vi "MicroscopeActor.vi"(8 "error in (no error)":errorcluster) -> (0 "error out":errorcluster)   [LabVIEW 2017]
doc: "Use this template to build a VI to use as a subVI."
uses:
  Spectrometer Utilities/SpectrometerCallbackdataEvent.ctl
  Microscope/MicroscopeControllerCluster.ctl
  <vilib>/vision/Image Controls.llb/IMAQ Image.ctl
  Microscope/MicroscopeActorCluster.ctl
  Database/DatabaseContollerGFVenum.ctl
  Microscope/MicroscopeControllerEnum.ctl
  <vilib>/userdefined/High Color/IMAQdx.ctl
  <vilib>/vision/driver/IMAQdx.llb/IMAQdx Camera Control Mode.ctl
  <vilib>/event_ctls.llb/lveventtype.ctl
  <vilib>/vision/NI_Vision_Development_Module.lvlib
  <vilib>/vision/driver/NI_Vision_Acquisition_Software.lvlib
panel:
  in  "Microscope Objective":u16(ring) caption="Combo Box" items=["50x", "5x", "10x"]
  in  "micron/pixel":dbl=0.10791300237178802
  in  "user event out":refnum<user-event>
  in  "user event Callback":refnum<user-event>
  in  "Add Objective":bool
  in  "TabEncompassingEditPointsControls":enum32{"Page 2"}(tab)
  in  "Choose Points":enum32{"Edit map Points", "Edit Laser Point"}(radio)=enum."Edit Laser Point"
  in  "TabEncompassMapEditControls":enum32{"Page 2"}(tab)
  in  "UndoBtn":bool
  out "# Points Selected":i32
  in  "Point Spacing":dbl=1.0 min=0.5 max=1000.0 format="%#_g µm"
  in  "Clear Points":bool
  in  "Edit Points":bool
  in  "Edit Laser Position":bool
  in  "Edit Map Points":bool=TRUE
  in  "Which point to translate?":i32
  in  "stop":bool
  out "Microscope Image":T1(plugin-control)
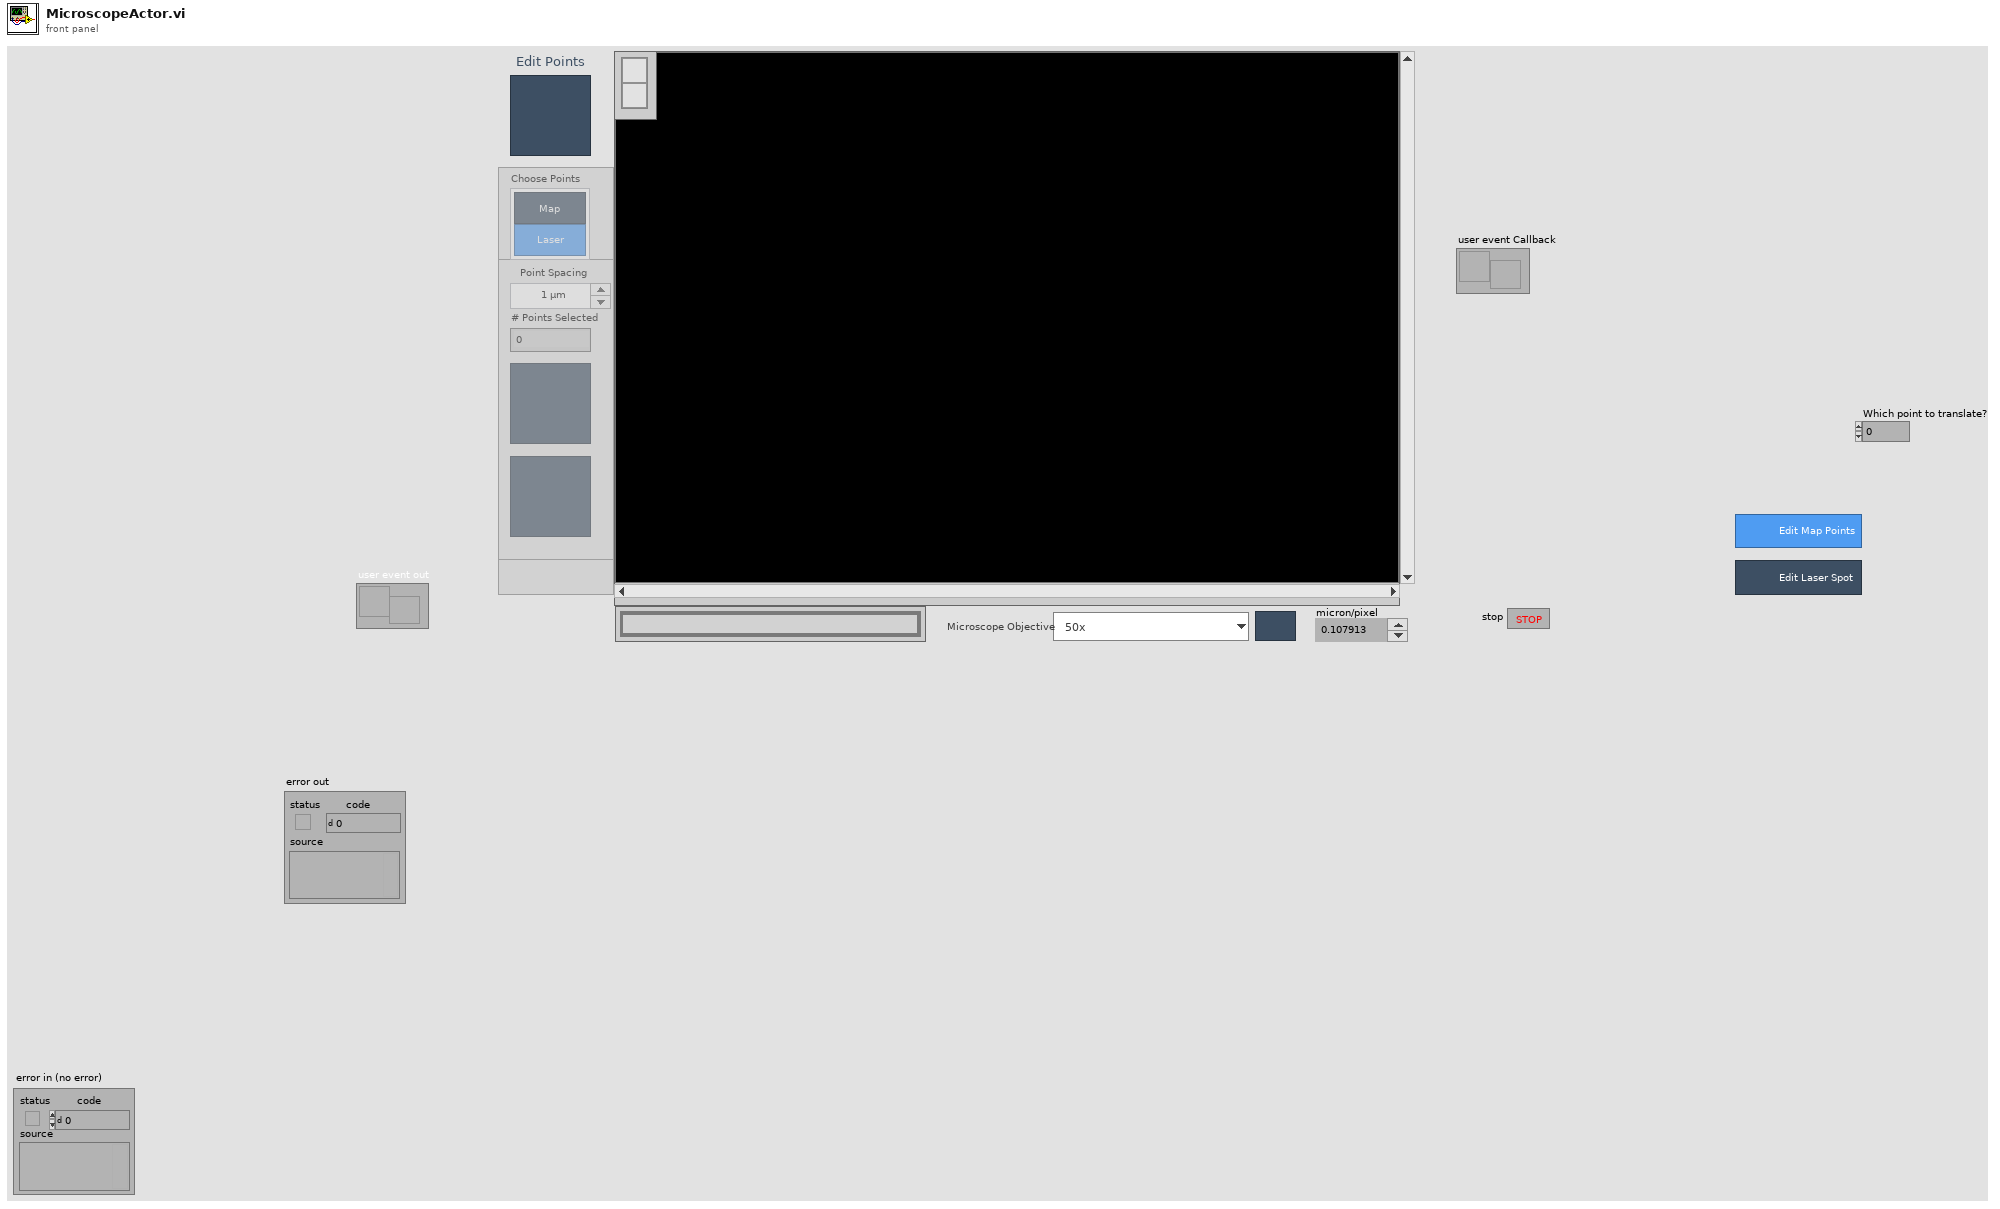
[diagram p1: front panel]
types:
  T1 = typedef "IMAQ Image.ctl" = refnum<image>
  T2 = typedef "Image Type" = u32
  T3 = typedef "DatabaseContollerGFVenum.ctl" = enum16{"Init and Open Database!", "GetTimeDifferencebetweenLastTwoMeasurements!", "Get next Journal Number!", "WriteInJournalTable", "GetNewMeas_dataIndex", "UpdateWithSpectrometerData", "UpdateWithMicroscopeData", "UpdateWithMapScriptData", "UpdateWithmainUIData", "Get Objective Microns/Pixels", "Get User Name!", "Get Active Users Names!", "Get User Picture!", "Get User Phone Number!", "Get Setup Names!", "Get Active Microscope Objectives!", "Get Experiment Number!", "Get Sample Types!", "Write meas_conf Table", "Write meas_data Table", "GetListOfIndices", "Get Objective Index", "Get last X Journal Entries"}
  T4 = typedef "MicroscopeControllerEnum.ctl" = enum16{"GetAllData!", "Init!", "Start!", "Stop!", "GetMicroscopeVIRef", "CalculateRelPointForStagemicrons", "InsertCallbackEvent!", "InsertLaserPoint!", "InsertMapPoints!", "InsertMicroscopeOverlayImageRef!", "GetMicroscopeOverlayImageRef", "InsertObjectiveIndex!", "InsertLiveImageRef", "GetLiveImageRef"}
  T5 = typedef "Image Unit" = enum32{"Undefined", "Angström", "Micrometer", "Millimeter", "Centimeter", "Meter", "Kilometer", "Microinch", "Inch", "Feet", "Nautical miles", "Standard miles", "Steps"}
  T6 = typedef "Simple Grid Descriptor" = cluster{"X Step":sgl, "Y Step":sgl, "Unit":T5}
  T7 = typedef "NI_Vision_Acquisition_Software.lvlib/IMAQdx Camera Control Mode.ctl" = enum32{"Controller", "Listener"}
  T8 = typedef "IMAQdx.ctl" = refnum<k21>
  T9 = typedef "MicroscopeActorCluster.ctl" = cluster{"Calibration Axis ":cluster{"Origin Pixel":cluster{"X":sgl, "Y":sgl}, "Angle Relative to Horizontal (deg)":sgl, "Axis Reference":u32}, "Microscope Image Overlay Ref":T1, "Laser Coordinate":cluster{"X":i32, "Y":i32}, "Map Points Coordinates":cluster{"X":i32, "Y":i32}[], "micron/pixel":dbl, "Microscope Image Live Ref":T1}
  T10 = cluster{"Origin Pixel":cluster{"X":sgl, "Y":sgl}, "Angle Relative to Horizontal (deg)":sgl, "Axis Reference":u32}
  T11 = typedef "MicroscopeControllerCluster.ctl" = cluster{"MapPointsArray":cluster{"X":i32, "Y":i32}[], "Laser Point Coor":cluster{"X":i32, "Y":i32}, "Microscope Image Overlay Ref":T1, "idObjectives":u32, "Microscope Image Live":T1}
  T12 = typedef "lveventtype.ctl" = enum32{"Null", "Timeout", "Annotation Menu Selection", "Annotation Menu Selection?", "App Instance Close", "App Instance Close?", "Autoscale Range Change", "Bookmark Info Change", "Cell Edit", "Cell Edit?", "Cursor Grab", "Cursor Grab?", "Cursor Menu Selection", "Cursor Menu Selection?", "Cursor Move", "Cursor Release", "Data Change", "Direction Change", "Display State Change", "Drag Ended", "Drag Enter", "Drag Leave", "Drag Over", "Drag Source Update", "Drag Starting", "Drag Starting?", "Drop", "Exec State Change", "Key Down", "Key Down?", "Key Repeat", "Key Repeat?", "Key Up", "Listbox Double Click", "Menu Activation?", "Menu Selection (App)", "Menu Selection? (App)", "Menu Selection (User)", "Mouse Down", "Mouse Down?", "Mouse Enter", "Mouse Leave", "Mouse Move", "Mouse Up", "Mouse Wheel", "NI Security User Change (App)", "Pane Size", "Panel Close", "Panel Close?", "Panel Resize", "Plot Attribute Change", "Scale Range Change", "Shortcut Menu Activation?", "Shortcut Menu Selection (App)", "Shortcut Menu Selection? (App)", "Shortcut Menu Selection (User)", "Tree Double Click", "Tree Drag", "Tree Drag?", "Tree Drop", "Tree Drop?", "Tree Item Close", "Tree Item Close?", "Tree Item Open", "Tree Item Open?", "User Event", "Value Change"}
  T13 = cluster{"Left":i32, "Top":i32, "Right":i32, "Bottom":i32}
  T14 = enum8{"Enabled", "Disabled", "Disabled and Grayed Out"}
  T15 = cluster{"Global Rectangle":i32[], "Contours":cluster{"Contour Type":u32, "ROI Type":u32, "Points":i32[]}[]}
  T16 = cluster{"Contour Type":u32, "ROI Type":u32, "Points":i32[]}[]
  T17 = cluster{"Contour Type":u32, "ROI Type":u32, "Points":i32[]}
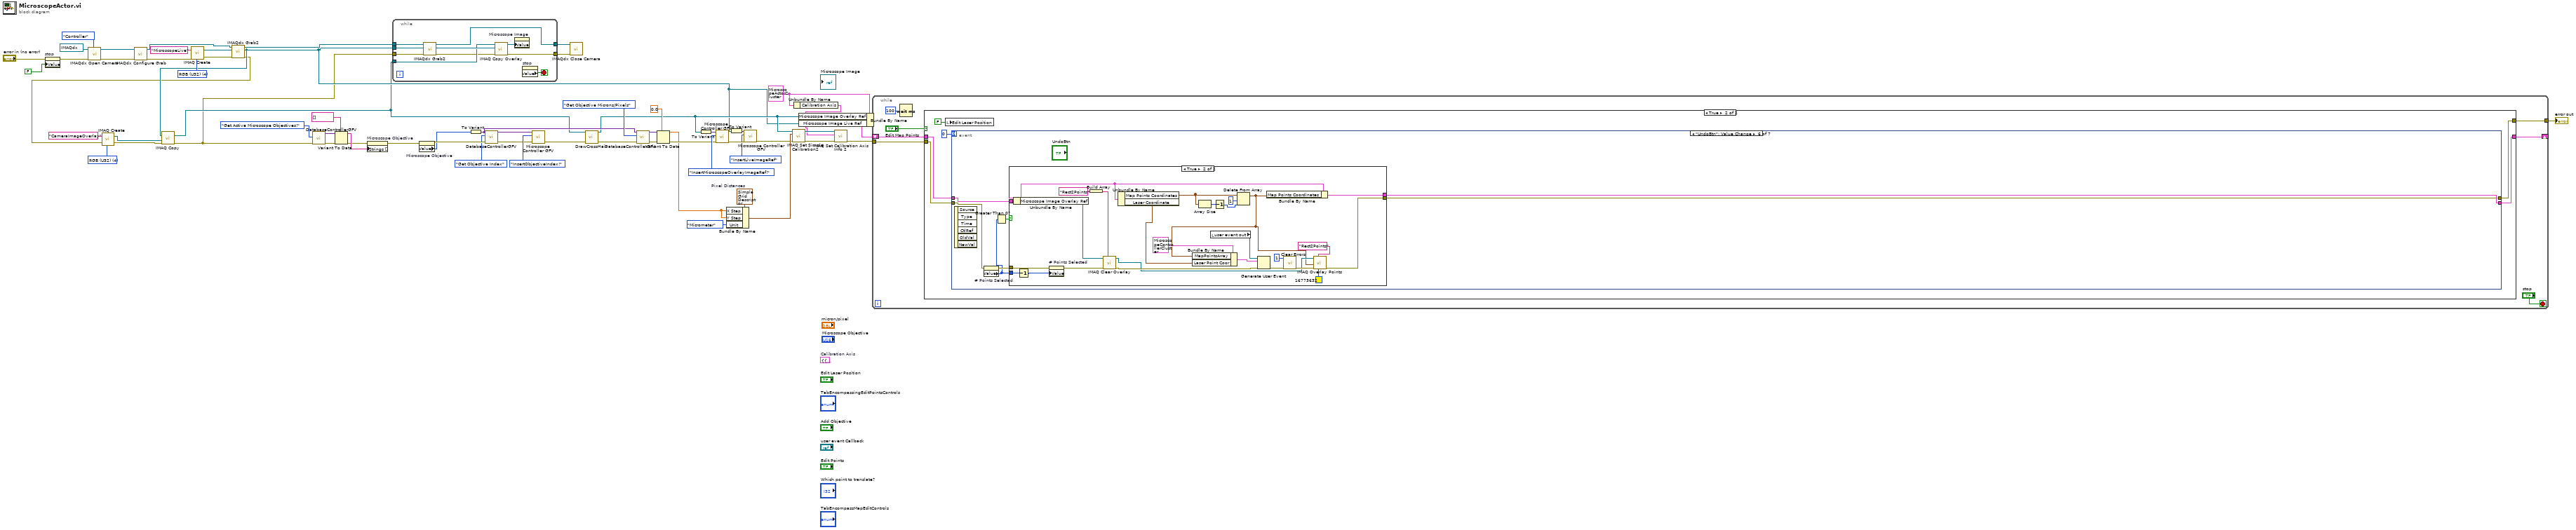
[diagram p0: block diagram]
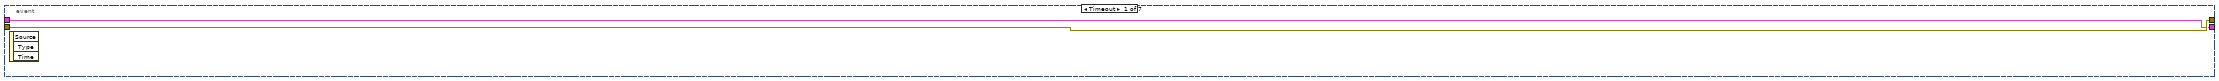
[diagram p3: hidden frame]
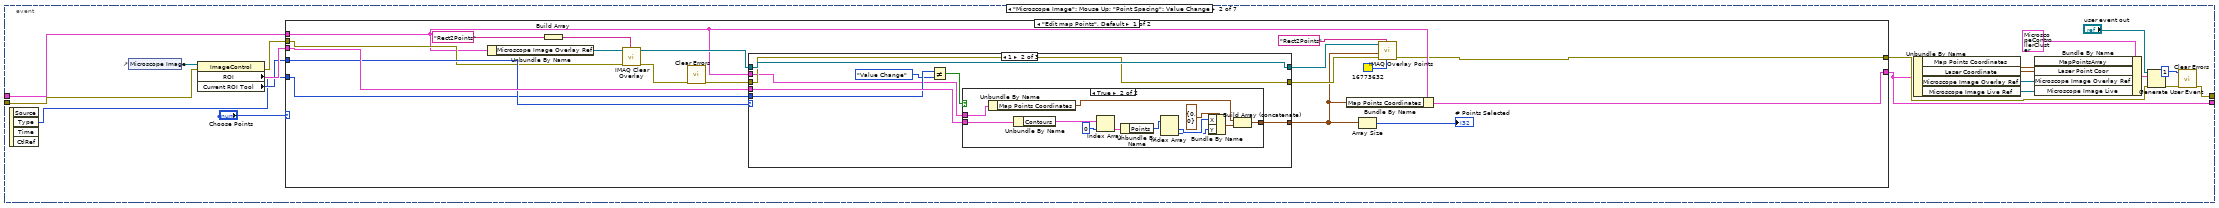
[diagram p4: hidden frame]
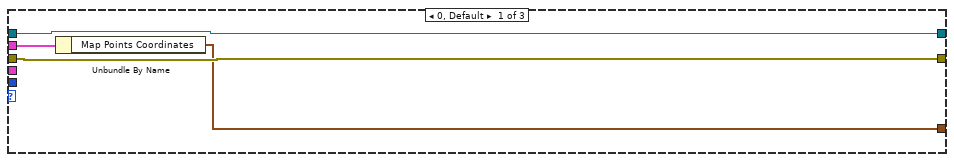
[diagram p5: hidden frame]
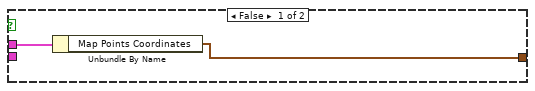
[diagram p6: hidden frame]
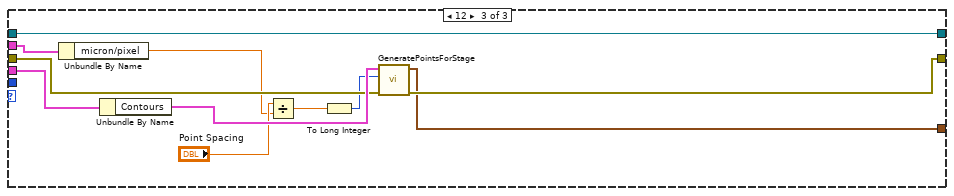
[diagram p7: hidden frame]
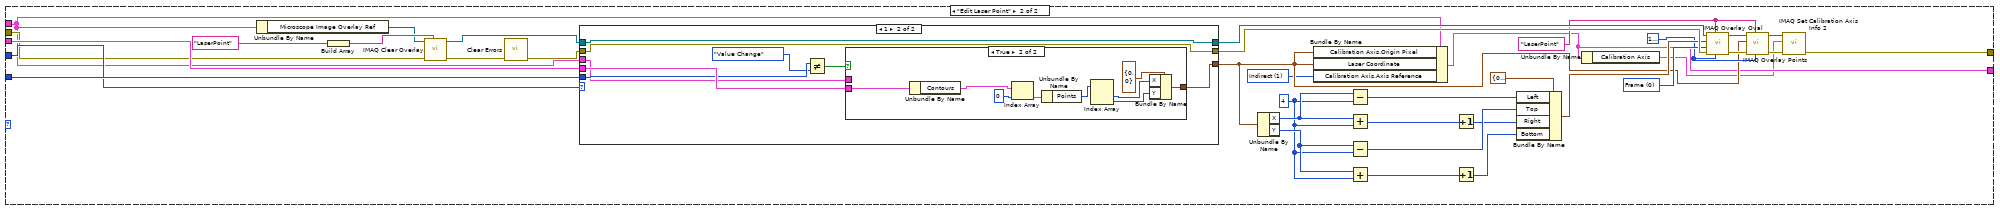
[diagram p8: hidden frame]
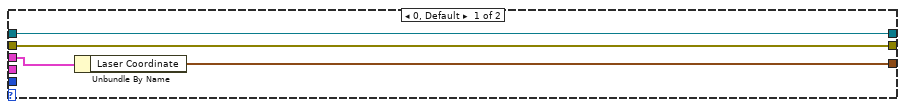
[diagram p9: hidden frame]
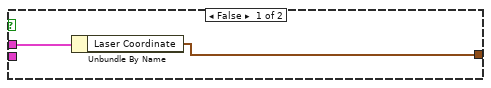
[diagram p10: hidden frame]
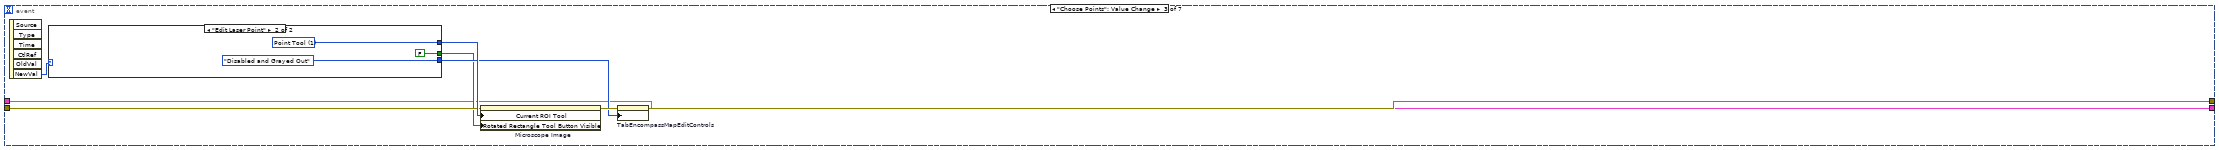
[diagram p11: hidden frame]
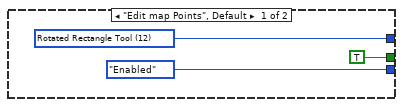
[diagram p12: hidden frame]
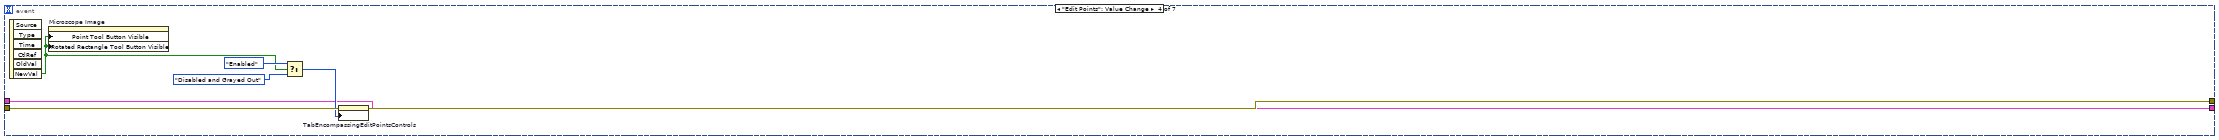
[diagram p13: hidden frame]
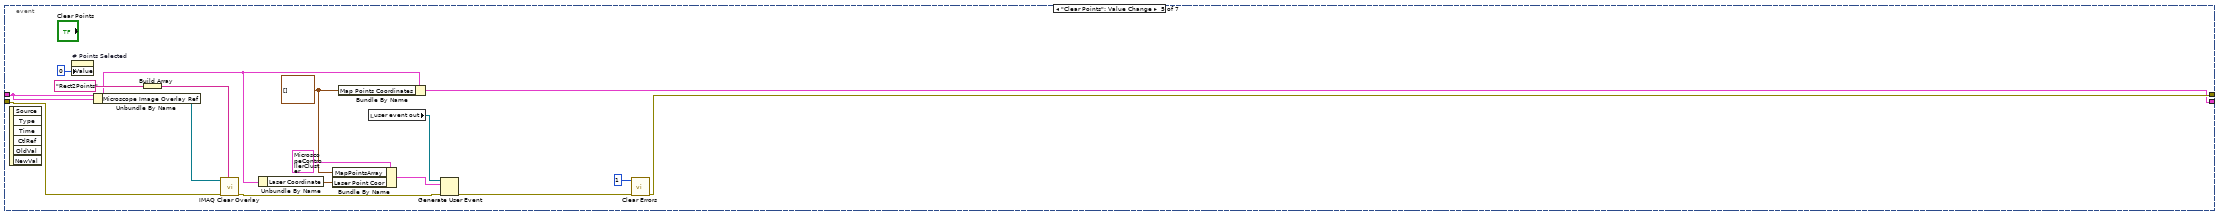
[diagram p14: hidden frame]
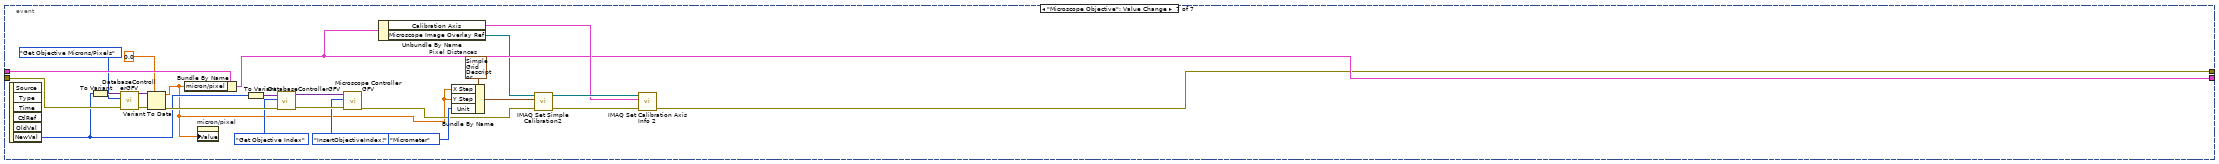
[diagram p16: hidden frame]
diagram:
  w15 = T2 4 items=["Grayscale (U8)", "Grayscale (I16)", "Grayscale (SGL)", "Complex (CSG)", "RGB (U32)", "HSL (U32)", "RGB (U64)", "Grayscale (U16)"] ("Image Type")
  w37 = T2 4 items=["Grayscale (U8)", "Grayscale (I16)", "Grayscale (SGL)", "Complex (CSG)", "RGB (U32)", "HSL (U32)", "RGB (U64)", "Grayscale (U16)"] ("Image Type")
  w45 = T6 {"X Step"=0.08029388, "Y Step"=0.08029388, "Unit"=enum."Micrometer"}  # Pixel Distances
  w39 = T9 {"Calibration Axis "={"Origin Pixel"={"X"=1232.0, "Y"=1028.0}, "Angle Relative to Horizontal (deg)"=0.0, "Axis Reference"=0}, "Microscope Image Overlay Ref"=refnum, "Laser Coordinate"={"X"=0, "Y"=0}, "Map Points Coordinates"=[], "micron/pixel"=0.10791300237178802, "Microscope Image Live Ref"=refnum}
  (unwired) T10 {"Origin Pixel"={"X"=1232.0, "Y"=1028.0}, "Angle Relative to Horizontal (deg)"=0.0, "Axis Reference"=0}  # Calibration Axis
  n1 = property on="stop" class="Bool (strict)"(error in="error in (no error)", "Value"=FALSE ("stop")) -> (error out=w3:errorcluster)  [unwired: 1 in, 1 out]
  n2 = call <vilib>:"IMAQdx Open Camera.vi"("Camera Control Mode"=IMAQdx_Camera_Control_Mode."Controller", "error in"=w3, "Session In"=T8 "cam2") -> ("error out"=w20:errorcluster, "Session Out"=w48:T8)  [unwired: 7 in]
  n3 = call <vilib>:"IMAQdx Configure Grab.vi"("error in"=w20, "Session In"=w48) -> ("error out"=w16:errorcluster, "Session Out"=w9:T8)  [unwired: 8 in]
  n4 = call "IMAQ Create"("Image Name"="MicroscopeLive", "Image Type"=w15, "error in (no error)"=w16) -> ("New Image"=w10:T1, "error out"=w11:errorcluster)  [unwired: 2 in]
  n5 = call <vilib>:"IMAQdx Grab2.vi"("error in"=w11, "Image In"=w10, "Session In"=w9) -> ("error out"=w2:errorcluster, "Image Out"=w5:T1, "Session Out"=w8:T8)  [unwired: 5 in, 1 out]
  n6 = call "IMAQ Create"("Image Name"="CameraImageOverlay", "Image Type"=w37, "error in (no error)"=w2) -> ("New Image"=w6:T1, "error out"=w7:errorcluster)  [unwired: 2 in]
  n7 = call "IMAQ Copy"("error in (no error)"=w7, "Image Dst"=w6, "Image Src"=w5) -> ("error out"=w1:errorcluster, "Image Dst Out"=w4:T1)  [unwired: 3 in]
  n8 = call "DatabaseControllerGFV.vi"("error in (no error)"=w1, "Enum"=DatabaseContollerGFVenum."Get Active Microscope Objectives!") -> ("error out"=w62:errorcluster, "Data Out"=w61:variant)  [unwired: 8 in]
  n9 = Variant To Data(error in=w62, type=string[] [], Variant=w61) -> (data=w59:string[], error out=w58:errorcluster)
  n10 = property on="Microscope Objective" class="Ring (strict)"(error in=w58, "Strings []"=w59) -> (error out=w52:errorcluster)  [unwired: 1 in, 1 out]
  n11 = while {
    tunnel: w8 -> [w73]
    tunnel: [w71] -> w19
    tunnel: [w70] -> w18
    tunnel: w5 -> [w72]
    tunnel: w4 -> [w67]
    tunnel: w1 -> [w64]
    stop <- w65 stop-if-true
    n12 = call <vilib>:"IMAQdx Grab2.vi"("error in"=w64, "Image In"=w72, "Session In"=w73) -> ("error out"=w66:errorcluster, "Image Out"=w69:T1, "Session Out"=w71:T8)  [unwired: 5 in, 1 out]
    n13 = call "IMAQ Copy Overlay"("error in (no error)"=w66, "Image Dst"=w69, "Image Src"=w67) -> ("error out"=w70:errorcluster, "Image Dst Out"=w68:T1)  [unwired: 7 in]
    n14 = property on="Microscope Image" class="ImageControl"("Value"=w68) -> ()  [unwired: 2 in, 2 out]
    n15 = property on="stop" class="Bool (strict)"() -> ("Value"=w65:bool)  [unwired: 2 in, 2 out]
  }
  n16 = property on="Microscope Objective" class="Ring (strict)"(error in=w52) -> (error out=w53:errorcluster, "Value"=w51:u16)  [unwired: 1 in, 1 out]
  n17 = To Variant(anything=w51) -> (Variant=w22:variant)
  n18 = call "DatabaseControllerGFV.vi"("error in (no error)"=w53, "Enum"=DatabaseContollerGFVenum."Get Objective Index", "Data in"=w22) -> ("error out"=w55:errorcluster, "Data Out"=w54:variant)  [unwired: 7 in]
  n19 = call "Microscope Controller GFV.vi"("error in (no error)"=w55, "MicroscopeEnum"=MicroscopeControllerEnum."InsertObjectiveIndex!", "Data in"=w54) -> ("error out"=w14:errorcluster)  [unwired: 7 in, 1 out]
  n20 = call <vilib>:"IMAQdx Close Camera.vi"("error in"=w18, "Session In"=w19) -> ()  [unwired: 9 in, 1 out]
  n21 = call "DrawCrossHair.vi"("error in (no error)"=w14, "Image In"=w4) -> ("error out"=w13:errorcluster, "Image Out"=w12:T1)  [unwired: 8 in]
  n22 = call "DatabaseControllerGFV.vi"("error in (no error)"=w13, "Enum"=DatabaseContollerGFVenum."Get Objective Microns/Pixels", "Data in"=w22) -> ("error out"=w26:errorcluster, "Data Out"=w23:variant)  [unwired: 7 in]
  n23 = Variant To Data(error in=w26, type=0.0 ("data"), Variant=w23) -> (data=w21:dbl, error out=w25:errorcluster)
  n24 = To Variant(anything=w12) -> (Variant=w30:variant)
  n25 = call "Microscope Controller GFV.vi"("error in (no error)"=w25, "MicroscopeEnum"=MicroscopeControllerEnum."InsertMicroscopeOverlayImageRef!", "Data in"=w30) -> ("error out"=w35:errorcluster)  [unwired: 7 in, 1 out]
  n26 = Bundle By Name(cluster=w45, "X Step"=w21, "Y Step"=w21, "Unit"=Image_Unit."Micrometer") -> (w43:T6)
  n27 = To Variant(anything=w5) -> (Variant=w31:variant)
  n28 = call "Microscope Controller GFV.vi"("error in (no error)"=w35, "MicroscopeEnum"=MicroscopeControllerEnum."InsertLiveImageRef", "Data in"=w31) -> ("error out"=w34:errorcluster)  [unwired: 7 in, 1 out]
  n29 = call "IMAQ Set Simple Calibration2"("error in (no error)"=w34, "Pixel Distances"=w43, "Image"=w12) -> ("error out"=w42:errorcluster, "Calibration Template Image"=w40:T1)  [unwired: 7 out]
  n30 = Unbundle By Name(w39) -> ("Calibration Axis"=w38:T10)
  n31 = Bundle By Name(cluster=w39, "Microscope Image Overlay Ref"=w12, "Microscope Image Live Ref"=w5) -> (w46:T9)
  n32 = call-poly "IMAQ Set Calibration Axis Info 2"("error in (no error)"=w42, "Calibration Axis Info"=w38, "Calibration Template Image In"=w40) -> ("error out"=w41:errorcluster)  [unwired: 7 in, 1 out]
  n33 = while {
    tunnel: [w79] -> w63
    tunnel: w41 -> [w78]
    shift-right: [w74] -> _
    shift-left: w46 -> [w75]
    stop <- "stop" stop-if-true
    n34 = Wait (ms)(milliseconds to wait=u32 100) -> ()  [unwired: 1 out]
    n35 = case shown="True" "Edit Map Points" {
      tunnel: [w82 w87] -> w79
      tunnel: w78 -> [w82 w86]
      tunnel: w75 -> [w81 w84]
      tunnel: [w81 w83] -> w74
      frame False {
      }
      frame True {
        n36 = local write "Edit Laser Position"(FALSE ("Edit Laser Position")) -> ()
        n37 = event shown="[5] \"UndoBtn\": Value Change" {
          selector: _ -> [_ _ _ _ _ _ _]
          dyn-events: _ -> [_ _ _ _ _ _ _]
          timeout: 0 -> [_ _ _ _ _ _ _]
          tunnel: [w90 w100 w229 w242 w254 w268 w298] -> w87
          tunnel: w86 -> [w90 w109 w231 w246 w262 w265 w316]
          tunnel: w84 -> [w89 w96 w226 w240 w248 w267 w322]
          tunnel: [w89 w95 w226 w240 w249 w269 w300] -> w83
          event Timeout {
            n38 = event-data() -> ()  [unwired: 1 in, 3 out]
          }
          event "Microscope Image": Mouse Up; "Point Spacing": Value Change {
            n39 = event-data() -> ("Type"=w106:T12)  [unwired: 1 in, 3 out]
            n40 = control-ref of="Microscope Image"() -> (w107:refnum<vi>)
            n41 = property class="ImageControl"(reference=w107, error in=w109) -> (error out=w104:errorcluster, "ROI"=w110:T15, "Current ROI Tool"=w108:u32)  [unwired: 1 out]
            n42 = case shown="\"Edit map Points\", Default" "Choose Points" {
              tunnel: w110 -> [w129 w201]
              tunnel: w108 -> [w128 w200]
              tunnel: w106 -> [w122 w202]
              tunnel: [w111 w167] -> w102
              tunnel: w104 -> [w121 w196]
              tunnel: w96 -> [w112 w175]
              tunnel: [w113 w171] -> w95
              frame "Edit map Points", Default {
                n43 = Unbundle By Name(w112) -> ("Microscope Image Overlay Ref"=w115:T1)
                n44 = Build Array("Rect2Points" ("Group")) -> (w118:string[])
                n45 = call "IMAQ Clear Overlay"("Groups"=w118, "error in (no error)"=w121, "Image"=w115) -> ("error out"=w117:errorcluster, "Image Out"=w120:T1)  [unwired: 7 in]
                n46 = call <vilib>:"Clear Errors.vi"("error in (no error)"=w117) -> ("error out"=w116:errorcluster)  [unwired: 5 in, 1 out]
                n47 = case shown="1" w128 {
                  tunnel: w129 -> [_ w141 w166]
                  tunnel: [w130 w140 w158] -> w114
                  tunnel: [w133 w139 w162] -> w124
                  tunnel: w116 -> [w132 w138 w164]
                  tunnel: w120 -> [w133 w139 w162]
                  tunnel: [w132 w138 w163] -> w126
                  tunnel: w122 -> [_ w137 _]
                  tunnel: w112 -> [w131 w134 w157]
                  frame 0, Default {
                    n48 = Unbundle By Name(w131) -> ("Map Points Coordinates"=w130:cluster{"X":i32, "Y":i32}[])
                  }
                  frame 1 {
                    n49 = Not Equal?(x=w137, y=lveventtype."Value Change" ("Type")) -> (x != y?=w135:bool)
                    n50 = case shown="True" w135 {
                      tunnel: w141 -> [_ w155]
                      tunnel: [w143 w145] -> w140
                      tunnel: w134 -> [w142 w144]
                      frame False {
                        n51 = Unbundle By Name(w142) -> ("Map Points Coordinates"=w143:cluster{"X":i32, "Y":i32}[])
                      }
                      frame True {
                        n52 = Unbundle By Name(w144) -> ("Map Points Coordinates"=w146:cluster{"X":i32, "Y":i32}[])
                        n53 = Unbundle By Name(w155) -> ("Contours"=w154:T16)
                        n54 = Index Array(array=w154, index=0) -> (element=w152:T17)
                        n55 = Unbundle By Name(w152) -> ("Points"=w150:i32[])
                        n56 = Index Array(array=w150) -> (element #1=w149:i32, element #2=w148:i32)  [unwired: 2 in]
                        n57 = Bundle By Name(cluster=cluster{"X":i32, "Y":i32} {"X"=0, "Y"=0} ("Point Coordinates"), "X"=w149, "Y"=w148) -> (w147:cluster{"X":i32, "Y":i32})
                        n58 = Build Array (concatenate)(w146, w147) -> (w145:cluster{"X":i32, "Y":i32}[])
                      }
                    }
                  }
                  frame 12 {
                    n59 = Unbundle By Name(w157) -> ("micron/pixel"=w156:dbl)
                    n60 = Unbundle By Name(w166) -> ("Contours"=w165:T16)
                    n61 = Divide(x="Point Spacing", y=w156) -> (x/y=w160:dbl)
                    n62 = To Long Integer(number=w160) -> (32bit integer=w159:i32)
                    n63 = call "GeneratePointsForStage.vi"("error in (no error)"=w164, "Point Spacing"=w159, "Rotated Rect"=w165) -> ("error out"=w163:errorcluster, "PointsInRotatedRect"=w158:cluster{"X":i32, "Y":i32}[])  [unwired: 7 in]
                  }
                }
                n64 = Bundle By Name(cluster=w112, "Map Points Coordinates"=w114) -> (w113:T9)
                n65 = Array Size(array=w114) -> (size(s)=→"# Points Selected":i32)
                n66 = call "IMAQ Overlay Points"("Color"=u32 16773632, "Group"="Rect2Points", "error in (no error)"=w126, "Array of Points"=w114, "Image"=w124) -> ("error out"=w111:errorcluster)  [unwired: 5 in, 1 out]
              }
              frame "Edit Laser Point" {
                w169 = u32 1 items=["Direct", "Indirect"] ("Axis Reference")
                w177 = 4 ("Laser Spot Size")
                w186 = u32 0 items=["Frame", "Fill"] ("Drawing Mode (Frame)")
                w183 = "LaserPoint" ("Group")
                w184 = u32 16777222 ("Color")
                n67 = Unbundle By Name(w175) -> ("Microscope Image Overlay Ref"=w176:T1)
                n68 = Build Array("LaserPoint" ("Group")) -> (w195:string[])
                n69 = call "IMAQ Clear Overlay"("Groups"=w195, "error in (no error)"=w196, "Image"=w176) -> ("error out"=w193:errorcluster, "Image Out"=w197:T1)  [unwired: 7 in]
                n70 = call <vilib>:"Clear Errors.vi"("error in (no error)"=w193) -> ("error out"=w192:errorcluster)  [unwired: 5 in, 1 out]
                n71 = case shown="1" w200 {
                  tunnel: w201 -> [_ w214]
                  tunnel: [w206 w213] -> w198
                  tunnel: w192 -> [w205 w212]
                  tunnel: w197 -> [w206 w213]
                  tunnel: [w205 w212] -> w199
                  tunnel: w202 -> [_ w211]
                  tunnel: [w203 w208] -> w174
                  tunnel: w175 -> [w204 w207]
                  frame 0, Default {
                    n72 = Unbundle By Name(w204) -> ("Laser Coordinate"=w203:cluster{"X":i32, "Y":i32})
                  }
                  frame 1 {
                    n73 = Not Equal?(x=w211, y=lveventtype."Value Change" ("Type")) -> (x != y?=w209:bool)
                    n74 = case shown="True" w209 {
                      tunnel: w214 -> [_ w225]
                      tunnel: [w215 w217] -> w208
                      tunnel: w207 -> [w216 _]
                      frame False {
                        n75 = Unbundle By Name(w216) -> ("Laser Coordinate"=w215:cluster{"X":i32, "Y":i32})
                      }
                      frame True {
                        n76 = Unbundle By Name(w225) -> ("Contours"=w224:T16)
                        n77 = Index Array(array=w224, index=0) -> (element=w222:T17)
                        n78 = Unbundle By Name(w222) -> ("Points"=w220:i32[])
                        n79 = Index Array(array=w220) -> (element #1=w219:i32, element #2=w218:i32)  [unwired: 2 in]
                        n80 = Bundle By Name(cluster=cluster{"X":i32, "Y":i32} {"X"=0, "Y"=0} ("Point Coordinates"), "X"=w219, "Y"=w218) -> (w217:cluster{"X":i32, "Y":i32})
                      }
                    }
                  }
                }
                n81 = Unbundle By Name(w174) -> ("X"=w188:i32, "Y"=w189:i32)
                n82 = Bundle By Name(cluster=w175, "Calibration Axis.Origin Pixel"=w174, "Laser Coordinate"=w174, "Calibration Axis.Axis Reference"=w169) -> (w171:T9)
                n83 = Subtract(x=w188, y=w177) -> (x-y=w190:i32)
                n84 = Add(x=w188, y=w177) -> (x+y=w178:i32)
                n85 = Subtract(x=w189, y=w177) -> (x-y=w182:i32)
                n86 = Add(x=w189, y=w177) -> (x+y=w181:i32)
                n87 = Increment(x=w178) -> (x+1=w179:i32)
                n88 = Increment(x=w181) -> (x+1=w180:i32)
                n89 = Bundle By Name(cluster=T13 {"Left"=0, "Top"=0, "Right"=0, "Bottom"=0} ("Bounding Rectangle"), "Left"=w190, "Top"=w182, "Right"=w179, "Bottom"=w180) -> (w187:T13)
                n90 = Unbundle By Name(w171) -> ("Calibration Axis"=w170:T10)
                n91 = call "IMAQ Overlay Oval"("Color"=w184, "Group"=w183, "error in (no error)"=w199, "Drawing Mode (Frame)"=w186, "Bounding Rectangle"=w187, "Image"=w198) -> ("error out"=w185:errorcluster, "Image Out"=w168:T1)  [unwired: 4 in]
                n92 = call "IMAQ Overlay Points"("Color"=w184, "Group"=w183, "error in (no error)"=w185, "Point"=w174, "Image"=w168) -> ("error out"=w173:errorcluster, "Image Out"=w172:T1)  [unwired: 5 in]
                n93 = call-poly "IMAQ Set Calibration Axis Info 2"("error in (no error)"=w173, "Calibration Axis Info"=w170, "Calibration Template Image In"=w172) -> ("error out"=w167:errorcluster)  [unwired: 7 in, 1 out]
              }
            }
            n94 = Unbundle By Name(w95) -> ("Map Points Coordinates"=w94:cluster{"X":i32, "Y":i32}[], "Laser Coordinate"=w93:cluster{"X":i32, "Y":i32}, "Microscope Image Overlay Ref"=w92:T1, "Microscope Image Live Ref"=w91:T1)
            n95 = Bundle By Name(cluster=T11 {"MapPointsArray"=[], "Laser Point Coor"={"X"=0, "Y"=0}, "Microscope Image Overlay Ref"=refnum, "idObjectives"=0, "Microscope Image Live"=refnum} ("event data"), "MapPointsArray"=w94, "Laser Point Coor"=w93, "Microscope Image Overlay Ref"=w92, "Microscope Image Live"=w91) -> (w97:T11)
            n96 = Generate User Event(user event="user event out", event data cluster=w97, error in=w102) -> (error out=w101:errorcluster)  [unwired: 1 in, 1 out]
            n97 = call <vilib>:"Clear Errors.vi"("error in (no error)"=w101, "specific error code to clear (0: all)"=1) -> ("error out"=w100:errorcluster)  [unwired: 4 in, 1 out]
          }
          event "Choose Points": Value Change {
            n98 = event-data() -> ("NewVal"=w233:enum32{"Edit map Points", "Edit Laser Point"})  [unwired: 1 in, 5 out]
            n99 = case shown="\"Edit Laser Point\"" w233 {
              tunnel: [w236 w239] -> w232
              tunnel: [T14."Enabled" ("Disabled") T14."Disabled and Grayed Out" ("Disabled")] -> w228
              tunnel: [TRUE ("ROI Tool Buttons Visible:Rotated Rectangle Tool Button Visible") FALSE ("ROI Tool Buttons Visible:Rotated Rectangle Tool Button Visible")] -> w227
              frame "Edit map Points", Default {
                w236 = u32 12 items=["Zoom Tool"=8, "Selection Tool"=0, "Pan Tool"=9, "Point Tool"=1, "Line Tool"=2, "Rectangle Tool"=3, "Rotated Rectangle Tool"=12, "Polyline Tool"=10, "Polygon Tool"=5, "Freehand Tool"=11, "Closed Freehand Tool"=6, "Ellipse Tool"=4, "Annulus Tool"=7] ("Current ROI Tool")
              }
              frame "Edit Laser Point" {
                w239 = u32 1 items=["Zoom Tool"=8, "Selection Tool"=0, "Pan Tool"=9, "Point Tool"=1, "Line Tool"=2, "Rectangle Tool"=3, "Rotated Rectangle Tool"=12, "Polyline Tool"=10, "Polygon Tool"=5, "Freehand Tool"=11, "Closed Freehand Tool"=6, "Ellipse Tool"=4, "Annulus Tool"=7] ("Current ROI Tool")
              }
            }
            n100 = property on="Microscope Image" class="ImageControl"(error in=w231, "Current ROI Tool"=w232, "Rotated Rectangle Tool Button Visible"=w227) -> (error out=w230:errorcluster)  [unwired: 1 in, 1 out]
            n101 = property on="TabEncompassMapEditControls" class="TabCtl (strict)"(error in=w230, "DisabledEnum"=w228) -> (error out=w229:errorcluster)  [unwired: 1 in, 1 out]
          }
          event "Edit Points": Value Change {
            n102 = event-data() -> ("NewVal"=w241:bool)  [unwired: 1 in, 5 out]
            n103 = property on="Microscope Image" class="ImageControl"("Point Tool Button Visible"=w241, "Rotated Rectangle Tool Button Visible"=w241) -> ()  [unwired: 2 in, 2 out]
            n104 = Select(t=T14."Enabled" ("Disabled"), s=w241, f=T14."Disabled and Grayed Out" ("Disabled")) -> (s? t:f=w243:T14)
            n105 = property on="TabEncompassingEditPointsControls" class="TabCtl (strict)"(error in=w246, "DisabledEnum"=w243) -> (error out=w242:errorcluster)  [unwired: 1 in, 1 out]
          }
          event "Clear Points": Value Change {
            w250 = cluster{"X":i32, "Y":i32}[] [] ("Shift points")
            n106 = event-data() -> ()  [unwired: 1 in, 6 out]
            n107 = property on="# Points Selected" class="DigNum (strict)"("Value"=0 ("Number of Points")) -> ()  [unwired: 2 in, 2 out]
            n108 = Unbundle By Name(w248) -> ("Microscope Image Overlay Ref"=w251:T1)
            n109 = Build Array("Rect2Points" ("Group")) -> (w259:string[])
            n110 = call "IMAQ Clear Overlay"("Groups"=w259, "error in (no error)"=w262, "Image"=w251) -> ("error out"=w255:errorcluster)  [unwired: 7 in, 1 out]
            n111 = Unbundle By Name(w248) -> ("Laser Coordinate"=w247:cluster{"X":i32, "Y":i32})
            n112 = Bundle By Name(cluster=T11 {"MapPointsArray"=[], "Laser Point Coor"={"X"=0, "Y"=0}, "Microscope Image Overlay Ref"=refnum, "idObjectives"=0, "Microscope Image Live"=refnum} ("event data"), "MapPointsArray"=w250, "Laser Point Coor"=w247) -> (w252:T11)
            n113 = Bundle By Name(cluster=w248, "Map Points Coordinates"=w250) -> (w249:T9)
            n114 = local read "user event out"() -> (w257:refnum<user-event>)
            n115 = Generate User Event(user event=w257, event data cluster=w252, error in=w255) -> (error out=w256:errorcluster)  [unwired: 1 in, 1 out]
            n116 = call <vilib>:"Clear Errors.vi"("error in (no error)"=w256, "specific error code to clear (0: all)"=1) -> ("error out"=w254:errorcluster)  [unwired: 4 in, 1 out]
          }
          event "UndoBtn": Value Change {
            n117 = event-data() -> ()  [unwired: 1 in, 6 out]
            n118 = property on="# Points Selected" class="DigNum (strict)"(error in=w265) -> (error out=w264:errorcluster, "Value"=w263:i32)  [unwired: 1 in, 1 out]
            n119 = Greater Than 0?(x=w263) -> (x > 0?=w266:bool)
            n120 = case shown="True" w266 {
              tunnel: w264 -> [w270 w278]
              tunnel: [w271 w289] -> w269
              tunnel: [w270 w284] -> w268
              tunnel: w267 -> [w271 w283]
              tunnel: w263 -> [_ w276]
              frame False {
              }
              frame True {
                n121 = Unbundle By Name(w283) -> ("Microscope Image Overlay Ref"=w290:T1)
                n122 = Decrement(x=w276) -> (x-1=w275:i32)
                n123 = property on="# Points Selected" class="DigNum (strict)"(error in=w278, "Value"=w275) -> (error out=w277:errorcluster)  [unwired: 1 in, 1 out]
                n124 = Build Array("Rect2Points" ("Group")) -> (w296:string[])
                n125 = call "IMAQ Clear Overlay"("Groups"=w296, "error in (no error)"=w277, "Image"=w290) -> ("error out"=w293:errorcluster, "Image Out"=w274:T1)  [unwired: 7 in]
                n126 = Unbundle By Name(w283) -> ("Map Points Coordinates"=w281:cluster{"X":i32, "Y":i32}[], "Laser Coordinate"=w272:cluster{"X":i32, "Y":i32})
                n127 = Array Size(array=w281) -> (size(s)=w280:i32)
                n128 = local read "user event out"() -> (w294:refnum<user-event>)
                n129 = Decrement(x=w280) -> (x-1=w279:i32)
                n130 = Delete From Array(array=w281, length=1, index=w279) -> (array with subset deleted=w273:cluster{"X":i32, "Y":i32}[])  [unwired: 1 out]
                n131 = Bundle By Name(cluster=T11 {"MapPointsArray"=[], "Laser Point Coor"={"X"=0, "Y"=0}, "Microscope Image Overlay Ref"=refnum, "idObjectives"=0, "Microscope Image Live"=refnum} ("event data"), "MapPointsArray"=w273, "Laser Point Coor"=w272) -> (w291:T11)
                n132 = Generate User Event(user event=w294, event data cluster=w291, error in=w293) -> (error out=w286:errorcluster)  [unwired: 1 in, 1 out]
                n133 = Bundle By Name(cluster=w283, "Map Points Coordinates"=w273) -> (w289:T9)
                n134 = call <vilib>:"Clear Errors.vi"("error in (no error)"=w286, "specific error code to clear (0: all)"=1) -> ("error out"=w285:errorcluster)  [unwired: 4 in, 1 out]
                n135 = call "IMAQ Overlay Points"("Color"=u32 16773632, "Group"="Rect2Points", "error in (no error)"=w285, "Array of Points"=w273, "Image"=w274) -> ("error out"=w284:errorcluster)  [unwired: 5 in, 1 out]
              }
            }
          }
          event "Microscope Objective": Value Change {
            w304 = T6 {"X Step"=0.08029388, "Y Step"=0.08029388, "Unit"=enum."Micrometer"}  # Pixel Distances
            n136 = event-data() -> ("NewVal"=w309:u16)  [unwired: 1 in, 5 out]
            n137 = To Variant(anything=w309) -> (Variant=w321:variant)
            n138 = call "DatabaseControllerGFV.vi"("error in (no error)"=w316, "Enum"=DatabaseContollerGFVenum."Get Objective Microns/Pixels", "Data in"=w321) -> ("error out"=w319:errorcluster, "Data Out"=w318:variant)  [unwired: 7 in]
            n139 = Variant To Data(error in=w319, type=0.0, Variant=w318) -> (data=w301:dbl, error out=w315:errorcluster)
            n140 = Bundle By Name(cluster=w322, "micron/pixel"=w301) -> (w300:T9)
            n141 = property on="micron/pixel" class="DigNum (strict)"("Value"=w301) -> ()  [unwired: 2 in, 2 out]
            n142 = To Variant(anything=w309) -> (Variant=w310:variant)
            n143 = call "DatabaseControllerGFV.vi"("error in (no error)"=w315, "Enum"=DatabaseContollerGFVenum."Get Objective Index", "Data in"=w310) -> ("error out"=w312:errorcluster, "Data Out"=w313:variant)  [unwired: 7 in]
            n144 = call "Microscope Controller GFV.vi"("error in (no error)"=w312, "MicroscopeEnum"=MicroscopeControllerEnum."InsertObjectiveIndex!", "Data in"=w313) -> ("error out"=w302:errorcluster)  [unwired: 7 in, 1 out]
            n145 = Unbundle By Name(w300) -> ("Calibration Axis"=w306:T10, "Microscope Image Overlay Ref"=w299:T1)
            n146 = Bundle By Name(cluster=w304, "X Step"=w301, "Y Step"=w301, "Unit"=Image_Unit."Micrometer") -> (w305:T6)
            n147 = call "IMAQ Set Simple Calibration2"("error in (no error)"=w302, "Pixel Distances"=w305, "Image"=w299) -> ("error out"=w307:errorcluster, "Calibration Template Image"=w308:T1)  [unwired: 7 out]
            n148 = call-poly "IMAQ Set Calibration Axis Info 2"("error in (no error)"=w307, "Calibration Axis Info"=w306, "Calibration Template Image In"=w308) -> ("error out"=w298:errorcluster)  [unwired: 7 in, 1 out]
          }
        }
      }
    }
  }
  "error out" <- w63
